vi "IV.vi"() -> ()   [LabVIEW 2016]
panel:
  in  "Repeats":i32=10
  out "Voltage":dbl format="%0.2f"
  out "Current":dbl format="%0.2f"
  in  "Initial V":dbl
  in  "Number of samples":i32=10
  in  "V Range":dbl
  in  "Range/N = dV":i32
  in  "Filename":path=path "C:/Users/tysoe-lab/Desktop/1.lvm"
  in  "Comment":string
  out "I/V Curve":cluster{"X":dbl[], "Y":dbl[]}[](graph) caption="XY Graph"
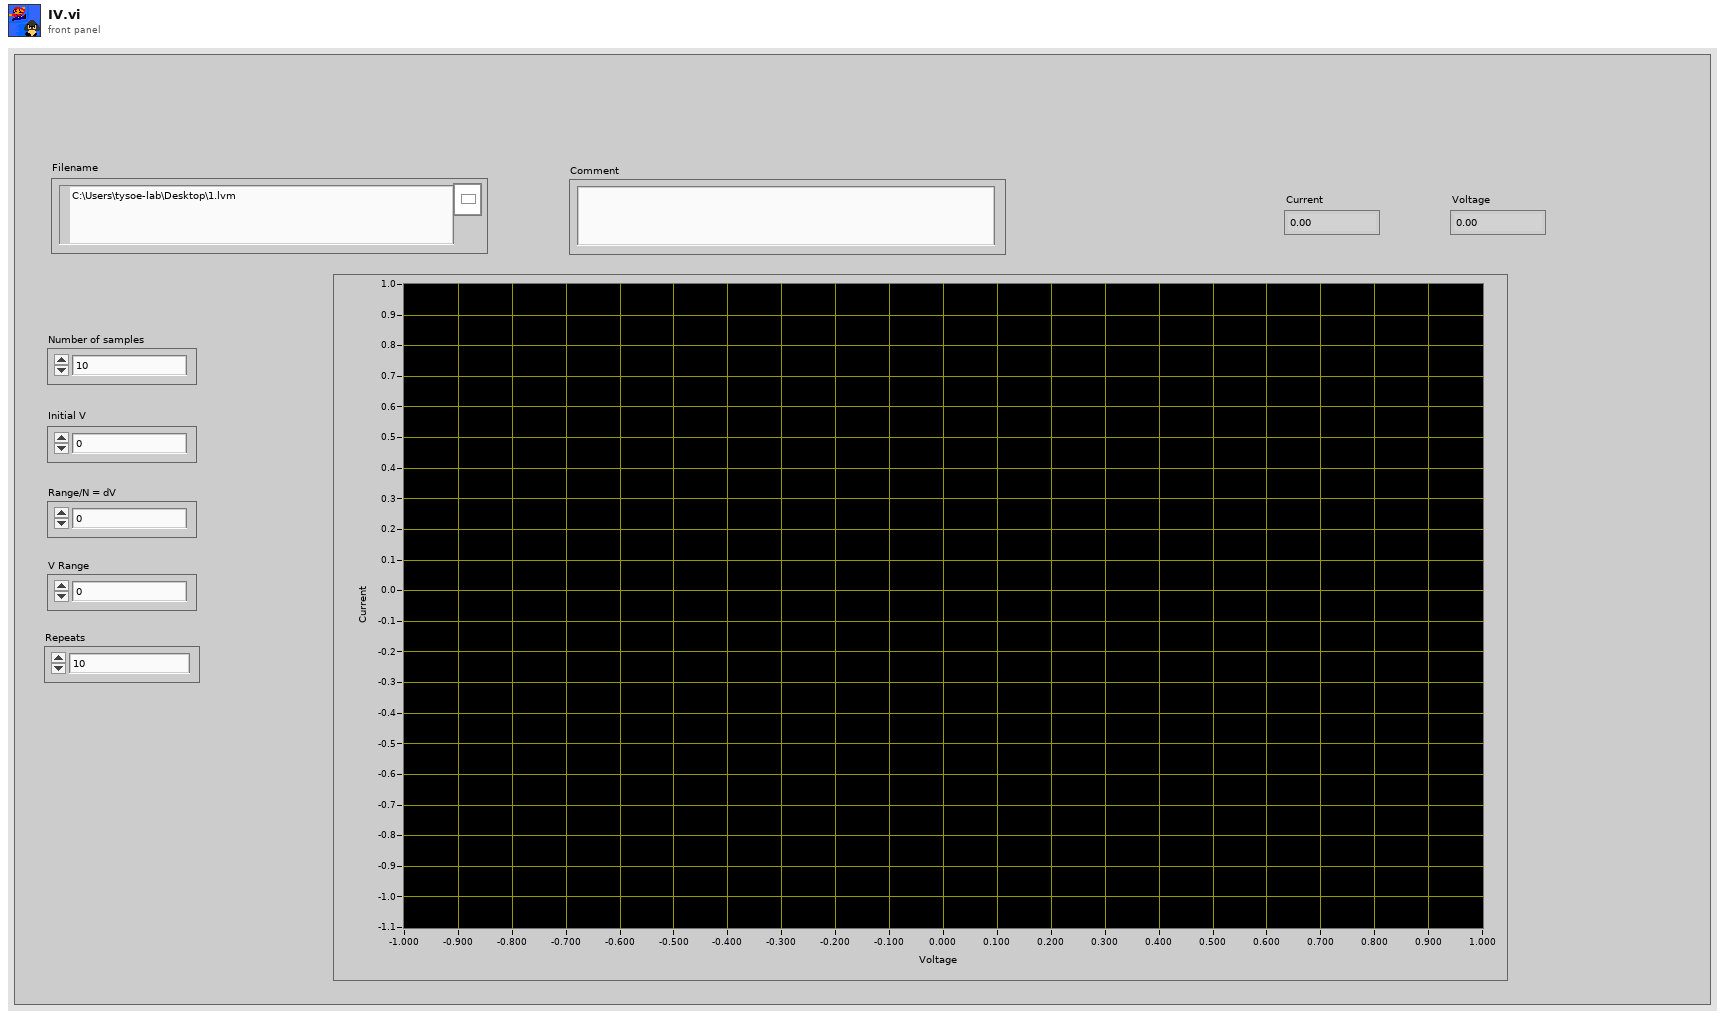
[diagram p1: front panel]
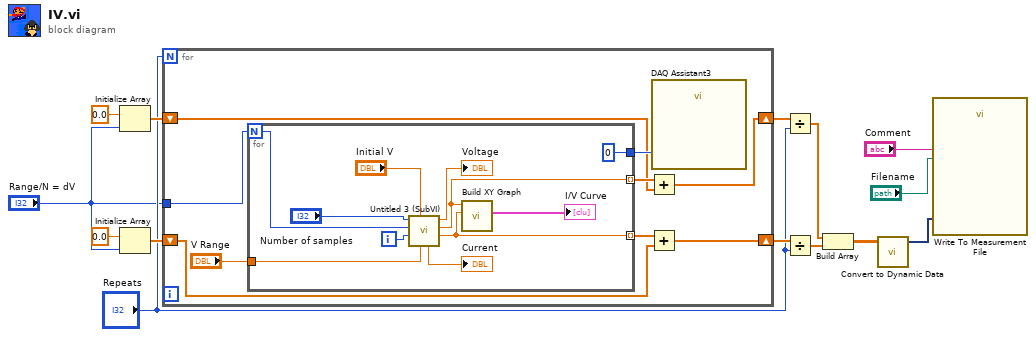
[diagram p0: block diagram]
diagram:
  n1 = Initialize Array(0.0 ("element"), "Range/N = dV") -> (w6:dbl[])
  n2 = Initialize Array(0.0 ("element"), "Range/N = dV") -> (w14:dbl[])
  n3 = for {
    N: "Repeats" -> [_]
    shift-right: [w19] -> w9
    shift-left: w14 -> [w21]
    shift-right: [w16] -> w5
    shift-left: w6 -> [w17]
    tunnel: "Range/N = dV" -> [w15]
    n4 = for {
      N: w15 -> [w30]
      tunnel: "V Range" -> [w32]
      tunnel: [w28] -> w20 mode=indexing
      tunnel: [w26] -> w18 mode=indexing
      tunnel: [0] -> w22
      i -> [w31]
      n5 = call "Untitled 3 (SubVI).vi"("V Range"=w32, "Initial V"="Initial V", "Numeric 3"=w31, "Numeric in"=w30, "Number of samples"="Number of samples") -> ("mean"=w28:dbl, "Numeric out"=w26:dbl, "Voltage"=→"Voltage":dbl, "Current"=→"Current":dbl)  [unwired: 3 in]
      n6 = call "Build XY Graph"("Y Input"=w28, "X Input"=w26) -> ("XY Graph"=→"I/V Curve":cluster{"X":dbl[], "Y":dbl[]}[])  [unwired: 8 in, 1 out]
    }
    n7 = Add(x=w18, y=w17) -> (x+y=w16:dbl[])
    n8 = Add(x=w20, y=w21) -> (x+y=w19:dbl[])
    n9 = call "DAQ Assistant3"("data"=w22) -> ()  [unwired: 17 in, 2 out]
  }
  n10 = Divide(x=w5, y="Repeats") -> (x/y=w4:dbl[])
  n11 = Divide(x=w9, y="Repeats") -> (x/y=w3:dbl[])
  n12 = Build Array(w4, w3) -> (w10:dbl[][])
  n13 = call "Convert to Dynamic Data"("2D Array"=w10) -> ("Dynamic Data Type"=w13:dynamicdata)  [unwired: 3 in]
  n14 = call "Write To Measurement File"("Signals"=w13, "Filename"="Filename", "Comment"="Comment") -> ()  [unwired: 14 in, 3 out]
